vi "Read Audio Data.vi"(8 "error in (no error)":errorcluster, 10 "Frames":u64, 11 "Channel in":refnum<data-value>) -> (0 "error out":errorcluster, 2 "Audio Data":dbl[][](array[numeric]), 3 "Channel out":refnum<data-value>)   [LabVIEW 2020, in "G-Audio.lvlib" / "Channel.lvclass"]
uses:
  Channel.lvclass
  Channel.lvclass/Channel.ctl
  Controls/Channel State.ctl
  <vilib>/Analysis/1siggen.llb/Ramp Pattern by Samples.vi
  <vilib>/Analysis/NI_AALBase.lvlib
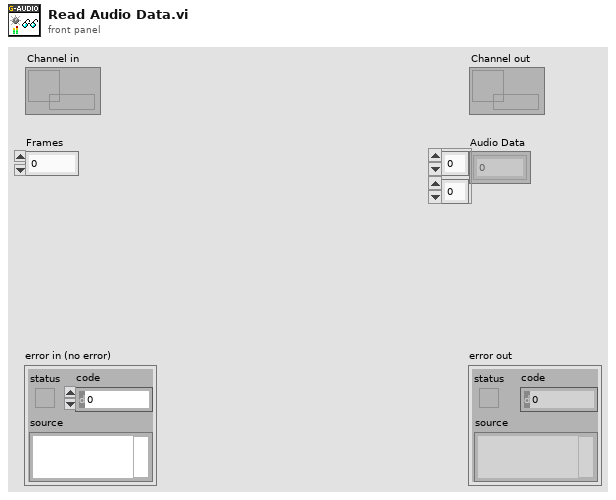
[diagram p1: front panel]
types:
  T1 = typedef "G-Audio.lvlib/Channel.lvclass/Channel State.ctl" = enum16{"Empty", "Loading", "Stopped", "Paused", "Playing", "Retrigger"}
  T2 = typedef "G-Audio.lvlib/Mixer.lvclass/Mixer Audio Data Type.ctl" = i16[][]
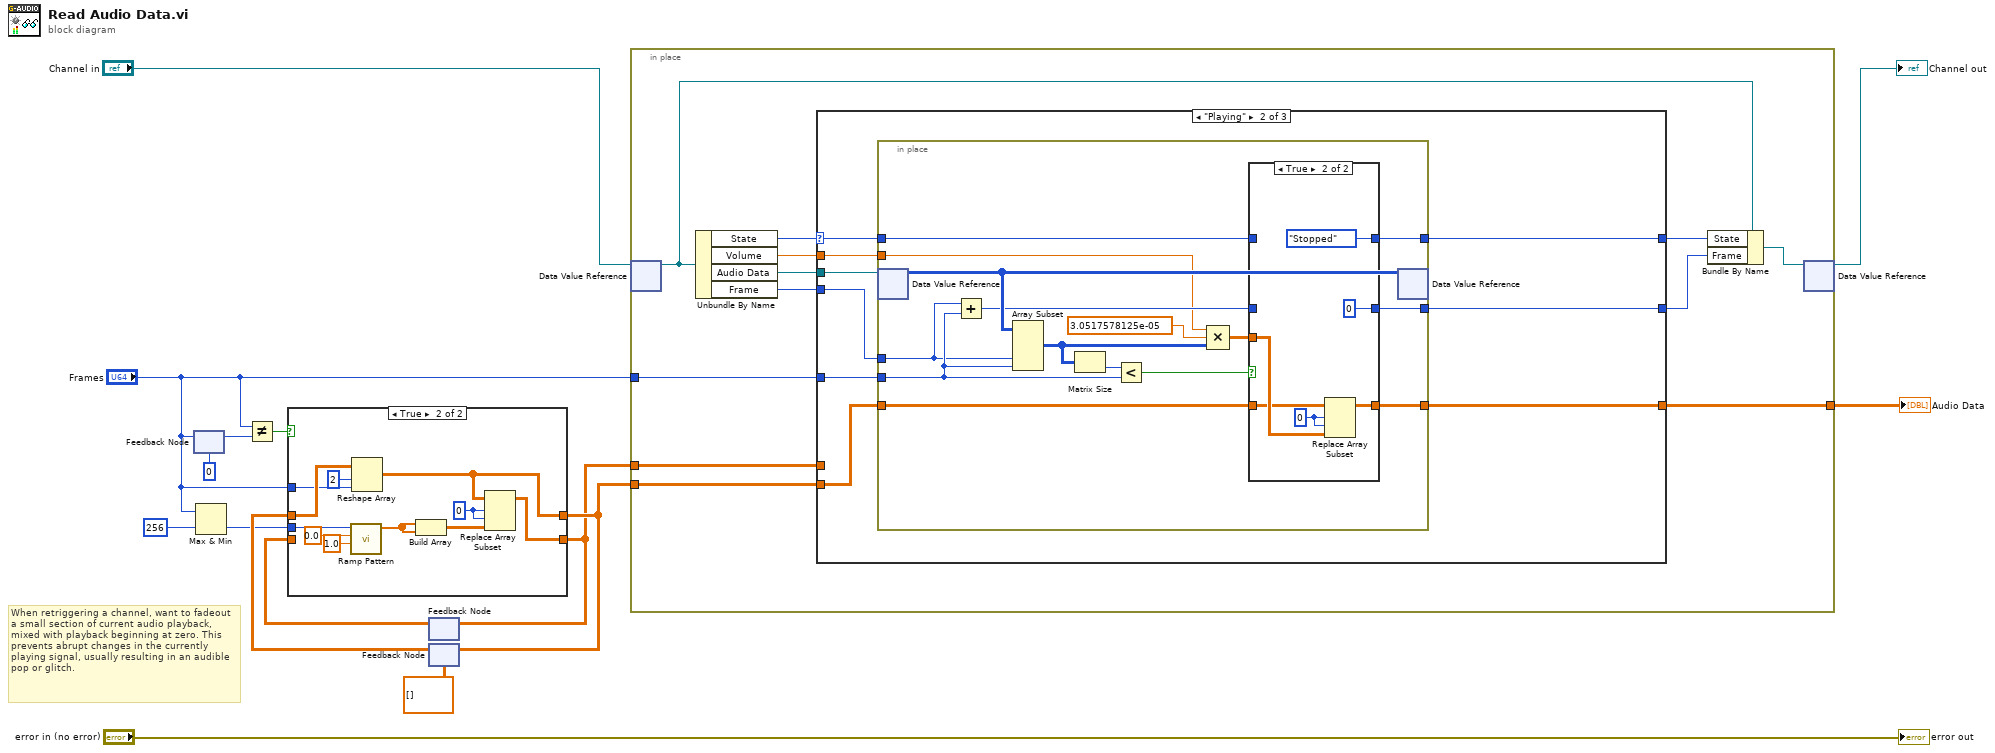
[diagram p0: block diagram]
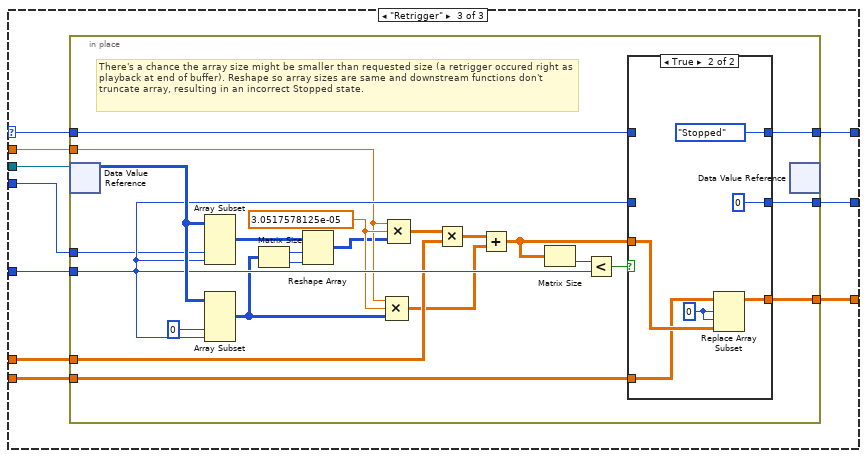
[diagram p5: hidden frame]
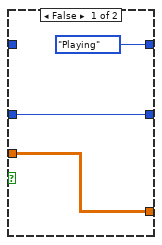
[diagram p6: hidden frame]
diagram:
  # "When retriggering a channel, want to fadeout a small section of current audio playback, mixed with playback beginning at zero. This prevents abrupt changes in the currently playing signal, usually resulting in an audible pop or glitch."
  n1 = feedback #1(u64 0 ("Frames")) -> (w14:u64)
  n2 = feedback-in #1("Frames") -> ()
  n3 = Max & Min(x="Frames", y=u64 256) -> (min(x,y)=w3:u64)  [unwired: 1 out]
  n4 = Not Equal?(x="Frames", y=w14) -> (x != y?=w13:bool)
  n5 = feedback #2() -> (w8:dbl[][])  [unwired: 1 in]
  n6 = feedback #3(dbl[][] [] ("Audio Data Type")) -> (w12:dbl[][])
  n7 = case shown="True" w13 {
    tunnel: "Frames" -> [_ w26]
    tunnel: [w17 w22] -> w11
    tunnel: w12 -> [w17 w28]
    tunnel: [w16 w19] -> w7
    tunnel: w8 -> [w16 _]
    tunnel: w3 -> [_ w23]
    frame False {
    }
    frame True {
      w21 = 0 ("index (row)")
      n8 = call-poly <vilib>:"Ramp Pattern.vi"("start"=1.0, "end"=0.0, "samples"=w23) -> ("Ramp Pattern"=w18:dbl[])  [unwired: 7 in, 1 out]
      n9 = Reshape Array(w28, u64 2 ("dimension size"), w26) -> (w22:dbl[][])
      n10 = Build Array(w18, w18) -> (w20:dbl[][])
      n11 = Replace Array Subset(array=w22, new element=w20, index (row)=w21, index (col)=w21) -> (w19:dbl[][])
    }
  }
  n12 = feedback-in #2(w7) -> ()
  n13 = feedback-in #3(w11) -> ()
  n14 = in-place {
    in-place-border: "Frames" -> [w40]
    in-place-border: [w39] -> w6
    in-place-border: w11 -> [w38]
    in-place-border: w7 -> [w37]
    n15 = in-place-dvr #4("Channel in") -> (w36:refnum<class "Channel.lvclass">)  [unwired: 1 out]
    n16 = Unbundle By Name(w36) -> ("State"=w31:T1, "Volume"=w32:dbl, "Audio Data"=w33:refnum<data-value>, "Frame"=w34:u64)
    n17 = case shown="\"Playing\"" w31 {
      selector: w31 -> [w43 w48 w82]
      tunnel: w40 -> [_ w52 w86]
      tunnel: w33 -> [_ w51 w85]
      tunnel: w34 -> [w41 w45 w78]
      tunnel: [w42 w50 w84] -> w39
      tunnel: [w43 w47 w81] -> w30
      tunnel: w38 -> [w42 w49 w83]
      tunnel: w37 -> [_ _ w80]
      tunnel: w32 -> [_ w46 w79]
      tunnel: [w41 w44 w77] -> w29
      frame Default {
      }
      frame "Playing" {
        n18 = in-place {
          in-place-border: w52 -> [w65]
          in-place-border: [w63] -> w50
          in-place-border: w49 -> [w62]
          in-place-border: w48 -> [w60]
          in-place-border: [w59] -> w47
          in-place-border: w46 -> [w55]
          in-place-border: w45 -> [w54]
          in-place-border: [w53] -> w44
          n19 = in-place-dvr #5(w51) -> (w67:T2)  [unwired: 1 out]
          n20 = Add(x=w54, y=w65) -> (x+y=w61:u64)
          n21 = Array Subset(array=w67, index (col)=w54, length (col)=w65) -> (w57:T2)  [unwired: 2 in]
          n22 = Matrix Size(0:w57) -> (2:w66:i32)  [unwired: 1 out]
          n23 = Less?(x=w66, y=w65) -> (x < y?=w64:bool)
          n24 = Compound Arithmetic op=MULTIPLY(w55, 3.0517578125e-05, w57) -> (w56:dbl[][])
          n25 = case shown="True" w64 {
            tunnel: [w70 w74] -> w63
            tunnel: w56 -> [w70 w76]
            tunnel: w62 -> [_ w75]
            tunnel: w61 -> [w69 _]
            tunnel: [w69 u64 0] -> w53
            tunnel: w60 -> [w68 _]
            tunnel: [w68 Channel_State."Stopped" ("State")] -> w59
            frame False {
            }
            frame True {
              w73 = 0 ("index (row)")
              n26 = Replace Array Subset(array=w75, new element=w76, index (row)=w73, index (col)=w73) -> (w74:dbl[][])
            }
          }
          n27 = in-place-dvr #5(w67) -> ()  [unwired: 2 out]
        }
      }
      frame "Retrigger" {
        n28 = in-place {
          in-place-border: w86 -> [w102]
          in-place-border: [w107] -> w84
          in-place-border: w83 -> [w106]
          in-place-border: w82 -> [w105]
          in-place-border: [w104] -> w81
          in-place-border: w80 -> [w98]
          in-place-border: w79 -> [w93]
          in-place-border: w78 -> [w92]
          in-place-border: [w91] -> w77
          w94 = 3.0517578125e-05
          # "There's a chance the array size might be smaller than requested size (a retrigger occured right as playback at end of buffer). Reshape so array sizes are same and downstream functions don't truncate array, resulting in an incorrect Stopped state."
          n29 = in-place-dvr #6(w85) -> (w103:T2)  [unwired: 1 out]
          n30 = Array Subset(array=w103, index (col)=w92, length (col)=w102) -> (w100:T2)  [unwired: 2 in]
          n31 = Array Subset(array=w103, index (col)=0 ("index"), length (col)=w102) -> (w89:T2)  [unwired: 2 in]
          n32 = Matrix Size(0:w89) -> (1:w88:i32, 2:w87:i32)
          n33 = Reshape Array(w100, w88, w87) -> (w90:T2)
          n34 = Compound Arithmetic op=MULTIPLY(w93, w94, w89) -> (w96:dbl[][])
          n35 = Compound Arithmetic op=MULTIPLY(w93, w94, w90) -> (w99:dbl[][])
          n36 = Multiply(x=w99, y=w98) -> (x*y=w97:dbl[][])
          n37 = Add(x=w97, y=w96) -> (x+y=w95:dbl[][])
          n38 = Matrix Size(0:w95) -> (2:w109:i32)  [unwired: 1 out]
          n39 = Less?(x=w109, y=w102) -> (x < y?=w108:bool)
          n40 = case shown="True" w108 {
            tunnel: [w112 w116] -> w107
            tunnel: w95 -> [w112 w118]
            tunnel: w106 -> [_ w117]
            tunnel: w102 -> [w111 _]
            tunnel: [w111 u64 0] -> w91
            tunnel: w105 -> [_ _]
            tunnel: [Channel_State."Playing" ("State") Channel_State."Stopped" ("State")] -> w104
            frame False {
            }
            frame True {
              w115 = 0 ("index (row)")
              n41 = Replace Array Subset(array=w117, new element=w118, index (row)=w115, index (col)=w115) -> (w116:dbl[][])
            }
          }
          n42 = in-place-dvr #6() -> ()  [unwired: 1 in, 2 out]
        }
      }
    }
    n43 = Bundle By Name(cluster=w36, "State"=w30, "Frame"=w29) -> (w35:refnum<class "Channel.lvclass">)
    n44 = in-place-dvr #4(w35) -> (→"Channel out":refnum<data-value>)  [unwired: 1 out]
  }
  "Audio Data" <- w6
  "error out" <- "error in (no error)"
